vi "_GetPeakList.vi"(2 "Minimum Height (100)":dbl=100.0, 3 "Current Data":T2={"Scan#"=0, "Run Time (mS)"=0, "TIC X"=[], "TIC Y"=[], "MassRange"=[], "Fixed Mass (amu)"=1.0, "Method"={"StartT(mS)"=0, "#Cycles"=0, "PauseT(uS)"=0, "ScanType"=0, "Polarity"=0, "FixedMass"=0.0, "DelayT(mS)"=0, "Active Ch"=[], "Mass Range"=[]}} {"Method"."Mass Range"."Res" items=["High/High", "Medium/Medium", "Low/Low", "High/Medium", "High/Low", "Medium/High", "Medium/Low", "Low/High", "Low/Medium"]}) -> (1 "PeakList":T1[](array[typedef]))   [LabVIEW 2015]
uses:
  Type/_Current Data.ctl
  Type/_XML Expt.ctl
  Type/_XML Lens.ctl
  Type/_Mass Range Property.ctl
  Type/_Mass Range Parameters.ctl
  Type/_RT Res Type.ctl
  Type/_Peak Property.ctl
  Type/_Log Command.ctl
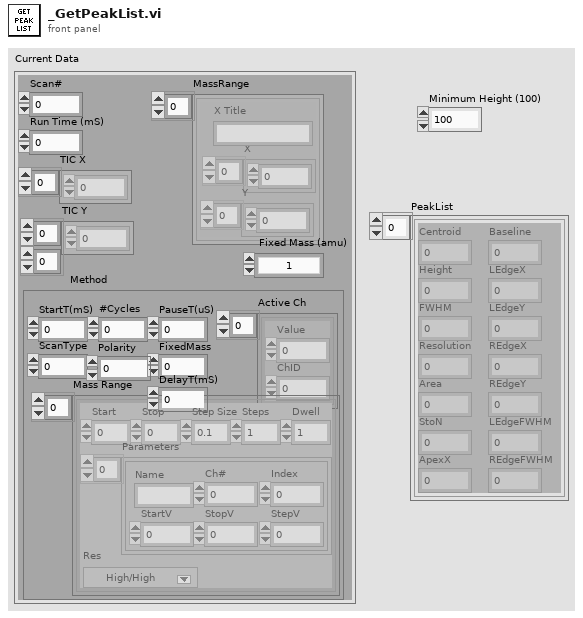
[diagram p1: front panel]
types:
  T1 = typedef "_Peak Property.ctl" = cluster{"Centroid":dbl, "Height":dbl, "FWHM":dbl, "Resolution":dbl, "Area":dbl, "StoN":dbl, "ApexX":dbl, "Baseline":dbl, "LEdgeX":dbl, "LEdgeY":dbl, "REdgeX":dbl, "REdgeY":dbl, "LEdgeFWHM":dbl, "REdgeFWHM":dbl}
  T2 = typedef "_Current Data.ctl" = cluster{"Scan#":i32, "Run Time (mS)":i32, "TIC X":dbl[], "TIC Y":dbl[][], "MassRange":cluster{"X Title":string, "X":dbl[], "Y":i32[]}[], "Fixed Mass (amu)":dbl, "Method":T3}
  T3 = typedef "_XML Expt.ctl" = cluster{"StartT(mS)":i32, "#Cycles":i32, "PauseT(uS)":i32, "ScanType":i32, "Polarity":u8, "FixedMass":dbl, "DelayT(mS)":i32, "Active Ch":T4[], "Mass Range":T5[]}
  T4 = typedef "_XML Lens.ctl" = cluster{"Value":dbl, "ChID":u8}
  T5 = typedef "_Mass Range Property.ctl" = cluster{"Start":dbl, "Stop":dbl, "Step Size":dbl, "Steps":i32, "Dwell":dbl, "Parameters":T6[], "Res":T7}
  T6 = typedef "_Mass Range Parameters.ctl" = cluster{"Name":string, "Ch#":u8, "StartV":dbl, "StopV":dbl, "StepV":dbl, "Index":u8}
  T7 = typedef "_RT Res Type.ctl" = u16
  T8 = cluster{"X Title":string, "X":dbl[], "Y":i32[]}[]
  T9 = typedef "_Log Command.ctl" = enum16{"No Command", "Open", "Read", "Write", "Close", "Check Size"}
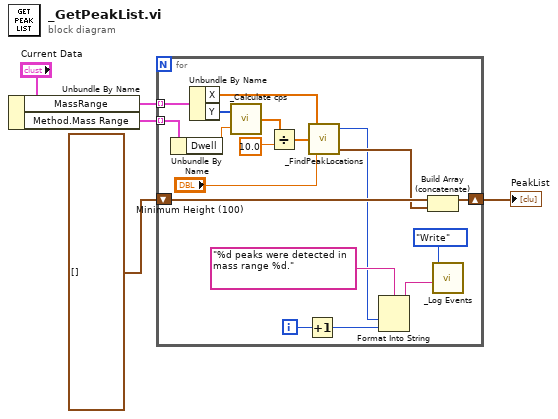
[diagram p0: block diagram]
diagram:
  n1 = Unbundle By Name("Current Data") -> ("MassRange"=w4:T8, "Method.Mass Range"=w1:T5[])
  n2 = for {
    tunnel: w4 -> [w23] mode=indexing
    shift-right: [w21] -> w2
    shift-left: T1[] [] ("Peak List") -> [w22]
    tunnel: w1 -> [w20] mode=indexing
    i -> [w15]
    n3 = Unbundle By Name(w20) -> ("Dwell"=w19:dbl)
    n4 = Unbundle By Name(w23) -> ("X"=w10:dbl[], "Y"=w18:i32[])
    n5 = call "_Calculate cps.vi"("Dwell (mS)"=w19, "Raw Counts"=w18) -> ("Data in cps"=w17:dbl[])
    n6 = Divide(x=w17, y=10.0) -> (x/y=w9:dbl[])
    n7 = Increment(x=w15) -> (x+1=w14:i32)
    n8 = call "_FindPeakLocations.vi"("threshold"="Minimum Height (100)", "Intensities"=w9, "Masses"=w10) -> ("Peak List"=w7:T1[], "# found"=w6:i32)  [unwired: 1 in]
    n9 = Format Into String(format string="%d peaks were detected in mass range %d." ("Event"), w6, w14) -> (resulting string=w12:string)  [unwired: 2 in, 1 out]
    n10 = Build Array (concatenate)(w22, w7) -> (w21:T1[])
    n11 = call "_Log Events.vi"("Event"=w12, "Log Command"=_Log_Command."Write") -> ()  [unwired: 6 in, 2 out]
  }
  "PeakList" <- w2
